vi "Global_Var_Drive.vi"() -> ()   [LabVIEW 2016]
panel:
  out "Extra_Motor_3":bool
  out "Extra_Motor_2":bool
  out "Extra_Motor_1":bool
  out "Left_Trigger":bool
  out "Right_Trigger":bool
  in  "Right_Joystick_Y":dbl
  in  "Left_Joystick_Y":dbl
  in  "Right_Joystick_X":dbl
  in  "Left_Joystick_X":dbl
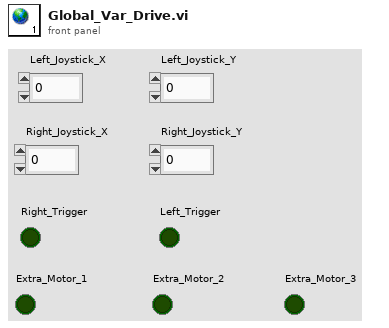
[diagram p1: front panel]
diagram:
